vi "随机数发生器（指数分布）.vi"(0 "n":i32=128, 1 "L":dbl=1.0) -> (4 "Random":dbl[](array[numeric]))   [LabVIEW 2011]
doc: "功能：\n\n产生指数分布的随机数\n\n\ncsxcs_366创建"
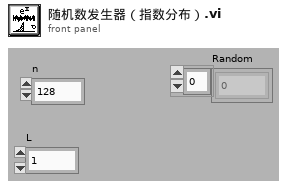
[diagram p1: front panel]
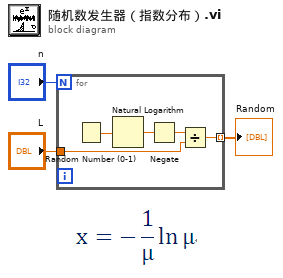
[diagram p0: block diagram]
diagram:
  n1 = for {
    N: "n" -> [_]
    tunnel: "L" -> [w5]
    tunnel: [w4] -> w1 mode=indexing
    n2 = Random Number (0-1)() -> (number: 0 to 1=w8:dbl)
    n3 = Natural Logarithm(1:w8) -> (0:w7:dbl)
    n4 = Negate(x=w7) -> (-x=w6:dbl)
    n5 = Divide(x=w6, y=w5) -> (x/y=w4:dbl)
  }
  "Random" <- w1
